vi "GetSuccessors.vi"(8 "error in (no error)":errorcluster, 10 "AbstractMapNode Ref":refnum<data-value>, 11 "WorldMap in":refnum<class "NI_Robotics_AbstractWorldMap.lvclass">) -> (0 "error out":errorcluster, 1 "EdgeCost":dbl[](array[numeric]), 2 "Successors":refnum<data-value>[](array[refnum]), 3 "WorldMap out":refnum<class "NI_Robotics_AbstractWorldMap.lvclass">)   [LabVIEW 2017, in "NI_Robotics_AbstractWorldMap.lvclass"]
uses:
  <vilib>/robotics/Navigation/shared/WorldMap/AbstractWorldMap/NI_Robotics_AbstractWorldMap.lvclass
  <vilib>/robotics/Navigation/shared/MapNode/AbstractMapNode/NI_Robotics_AbstractMapNode.lvclass
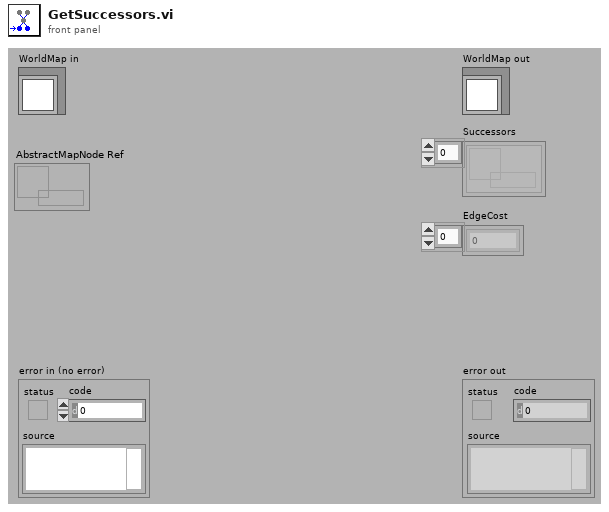
[diagram p1: front panel]
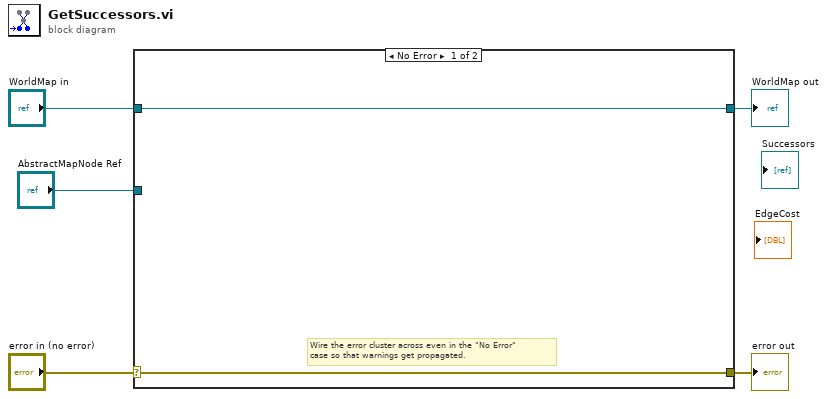
[diagram p0: block diagram]
diagram:
  n1 = case shown="No Error" "error in (no error)" {
    selector: "error in (no error)" -> [w6 w9]
    tunnel: [w6 w9] -> w4
    tunnel: [w7 w8] -> w2
    tunnel: "WorldMap in" -> [w7 w8]
    tunnel: "AbstractMapNode Ref" -> [_ _]
    frame No Error {
      # "Wire the error cluster across even in the \"No Error\"\ncase so that warnings get propagated."
    }
    frame Error {
    }
  }
  "error out" <- w4
  "WorldMap out" <- w2
